vi "Auto Drive.vi"(9 "Right Output":dbl, 10 "Left Output":dbl, 11 "Execute?":bool) -> (3 "Done":bool)   [LabVIEW 2012]
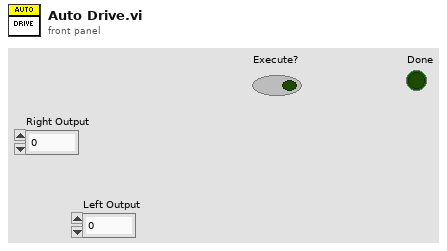
[diagram p1: front panel]
types:
  T1 = typedef "WPI_MotorControlDeviceRef.ctl" = cluster{"DeviceStatus":errorcluster, "Type":enum16{"PWM", "CAN"}, "PWM":cluster{"Digital Module":T2, "PWM Channel":T3, "DeadBand":T4}, "CAN":cluster{"Device Number":u8, "Control Mode":T5, "Semaphore":T6, "Max Vout":dbl}, "Invert":bool, "TransformRef":T7, "InvTransformRef":T7}
  T2 = typedef "FPGA_TypedefDigitalModule.ctl" = enum16{"Digital Module 1", "Digital Module 2"}
  T3 = typedef "FPGA_DIOPWMChannel.ctl" = enum8{"PWM 1", "PWM 2", "PWM 3", "PWM 4", "PWM 5", "PWM 6", "PWM 7", "PWM 8", "PWM 9", "PWM 10", "Invalid"}
  T4 = typedef "WPI_PWMDeadband.ctl" = cluster{"Name":string, "maxPositivePwm":i32, "minPositivePwm":i32, "centerPwm":i32, "maxNegativePwm":i32, "minNegativePwm":i32, "angularRange":u16}
  T5 = typedef "WPI_CANJaguar_ControlMode.ctl" = enum8{"Percent VBus", "Current", "Speed", "Position", "Voltage"}
  T6 = typedef "Semaphore RefNum" = refnum<k1>
  T7 = typedef "WPI_PWMTransform_ConPane.ctl" = refnum<vi>
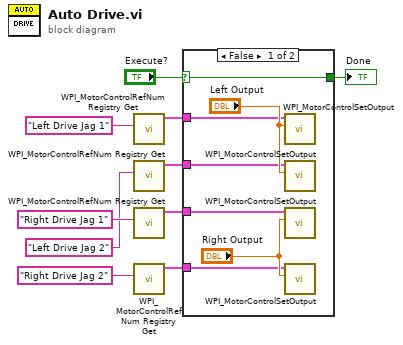
[diagram p0: block diagram]
diagram:
  n1 = call <vilib>:"WPI_MotorControlRefNum Registry Get.vi"("refnum name"="Left Drive Jag 1") -> ("MotorControlDevRef"=w4:T1)  [unwired: 9 in, 1 out]
  n2 = call <vilib>:"WPI_MotorControlRefNum Registry Get.vi"("refnum name"="Left Drive Jag 2") -> ("MotorControlDevRef"=w3:T1)  [unwired: 9 in, 1 out]
  n3 = call <vilib>:"WPI_MotorControlRefNum Registry Get.vi"("refnum name"="Right Drive Jag 1") -> ("MotorControlDevRef"=w2:T1)  [unwired: 9 in, 1 out]
  n4 = call <vilib>:"WPI_MotorControlRefNum Registry Get.vi"("refnum name"="Right Drive Jag 2") -> ("MotorControlDevRef"=w1:T1)  [unwired: 9 in, 1 out]
  n5 = case shown="False" "Execute?" {
    selector: "Execute?" -> [w17 w18]
    tunnel: [w17 w18] -> w9
    tunnel: w4 -> [w14 _]
    tunnel: w3 -> [w13 _]
    tunnel: w2 -> [w12 _]
    tunnel: w1 -> [w11 _]
    frame False {
      n6 = call <vilib>:"WPI_MotorControlSetOutput.vi"("Output"="Left Output", "MotorControlDevRef"=w14) -> ()  [unwired: 7 in, 3 out]
      n7 = call <vilib>:"WPI_MotorControlSetOutput.vi"("Output"="Left Output", "MotorControlDevRef"=w13) -> ()  [unwired: 7 in, 3 out]
      n8 = call <vilib>:"WPI_MotorControlSetOutput.vi"("Output"="Right Output", "MotorControlDevRef"=w12) -> ()  [unwired: 7 in, 3 out]
      n9 = call <vilib>:"WPI_MotorControlSetOutput.vi"("Output"="Right Output", "MotorControlDevRef"=w11) -> ()  [unwired: 7 in, 3 out]
    }
    frame True {
    }
  }
  "Done" <- w9
